vi "original_config.vi"() -> ()   [LabVIEW 2019]
uses:
  RT/RT Controls/Main Box Config.ctl
  <vilib>/Utility/config.llb/Read Key (String).vi
  <vilib>/Utility/config.llb/NI_LVConfig.lvlib
panel:
  out "value":T1={"WatchdogTim"=600, "DirRevDel"=4, "Coast"=0.5, "HSThres"=5.0, "EncCounts360"=4018143232, "HomePos"=0.0, "EncRefDeg"=0.0, "EncRefCounts"=79895940197, "Tol"=1.0, "CloudEn"=FALSE, "AutoShutEn"=FALSE, "RainTim"=5, "AZTimeout"=120, "AZEncPol"=enum."Positive"} {"Tol" format="%.2f"; "EncRefDeg" format="%.2f"; "HomePos" format="%.2f"; "HSThres" format="%.2f"; "Coast" format="%.2f"}
  out "error out":errorcluster
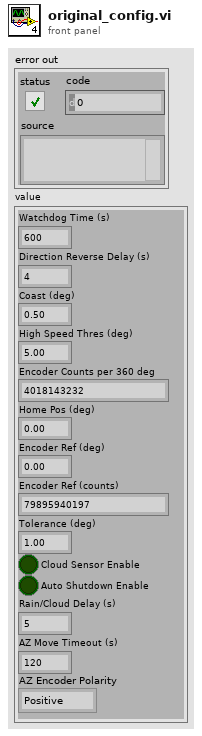
[diagram p1: front panel]
types:
  T1 = typedef "Main Box Config.ctl" = cluster{"WatchdogTim":i32, "DirRevDel":i32, "Coast":dbl, "HSThres":dbl, "EncCounts360":u64, "HomePos":dbl, "EncRefDeg":dbl, "EncRefCounts":u64, "Tol":dbl, "CloudEn":bool, "AutoShutEn":bool, "RainTim":i32, "AZTimeout":i32, "AZEncPol":enum16{"Positive", "Negative"}}
  T2 = typedef "NI_LVConfig.lvlib/Config Data RefNum.ctl" = refnum<k1>
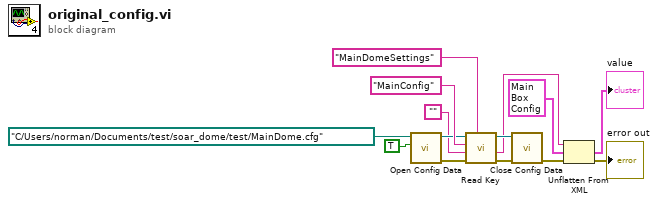
[diagram p0: block diagram]
diagram:
  n1 = call <vilib>:"Open Config Data.vi"("create file if necessary (T)"=TRUE, "configuration file path"=path "C:/Users/norman/Documents/test/soar_dome/test/MainDome.cfg") -> ("error out"=w10:errorcluster, "refnum"=w9:T2)  [unwired: 7 in, 1 out]
  n2 = call-poly <vilib>:"Read Key.vi"("section"="MainDomeSettings", "error in (no error)"=w10, "default value"="", "key"="MainConfig" ("section"), "refnum"=w9) -> ("error out"=w7:errorcluster, "value"=w5:string, "refnum out"=w8:T2)  [unwired: 3 in, 1 out]
  n3 = call <vilib>:"Close Config Data.vi"("error in (no error)"=w7, "refnum"=w8) -> ("error out"=w4:errorcluster)  [unwired: 8 in, 1 out]
  n4 = Unflatten From XML(xml string=w5, type=T1 {"WatchdogTim"=600, "DirRevDel"=5, "Coast"=0.0, "HSThres"=0.0, "EncCounts360"=0, "HomePos"=0.0, "EncRefDeg"=0.0, "EncRefCounts"=0, "Tol"=0.0, "CloudEn"=FALSE, "AutoShutEn"=FALSE, "RainTim"=5, "AZTimeout"=300, "AZEncPol"=enum."Positive"} ("MainBoxConfig"), error in (no error)=w4) -> (value=→"value":T1, error out=→"error out":errorcluster)
